vi "Test Customer Pick Up Order Broadcasts Status Update.vi"(8 "error in (no error)":errorcluster, 11 "Customer Test in":refnum<class "Customer Test.lvclass">) -> (0 "error out":errorcluster, 3 "Customer Test out":refnum<class "Customer Test.lvclass">)   [LabVIEW 2020, in "Customer Test.lvclass"]
uses:
  Customer Test.lvclass
  C:/Program Files (x86)/National Instruments/LabVIEW 2020/vi.lib/Asteme/LUnit/Test Case.lvclass
  Processes/People/Customers/Customer/Customer.lvclass
  C:/Program Files (x86)/National Instruments/LabVIEW 2020/vi.lib/Asteme/Triarc Framework/Process/Process.lvclass
  Support/Beverages/Beverage/Beverage.lvclass
  <vilib>/Asteme/LUnit/Test Case.lvclass/Test Case.ctl
  <vilib>/Asteme/LUnit/LUnit Assertion Result.lvclass/LUnit Assertion Result.ctl
  <vilib>/Asteme/Triarc Framework/Process/Process.lvclass/Process.ctl
  <vilib>/Asteme/Triarc Framework/Broadcast Event Helpers/Execution timer.vi
  <vilib>/Asteme/LUnit/Palette/Pass If.vi
  <vilib>/Asteme/LUnit/Set Assertion Type.vi
  <vilib>/Asteme/Triarc Framework/Process/Private/SubVIs/Wait for finish.vi
  <vilib>/Asteme/Triarc Framework/Process/Protected/Messaging/Enqueue Message.vi
  <vilib>/Asteme/Triarc Framework/Process/Private/SubVIs/Set Lifecycle State.vi
  <vilib>/Asteme/Triarc Framework/Process/Public/Lifecycle/Get Lifecycle State.vi
  <vilib>/Asteme/LUnit/Palette/Fail.vi
  <vilib>/Asteme/LUnit/Palette/Pass.vi
  <vilib>/Asteme/LUnit/LUnit Write Assertion Type.vi
  <vilib>/Asteme/LUnit/Add test result.vi
  <vilib>/Asteme/LUnit/LUnit Write Passed.vi
  <vilib>/Asteme/LUnit/LUnit Get Test Case.vi
  <vilib>/Asteme/LUnit/Assertion Result/LUnit Get Test Name.vi
  <vilib>/Asteme/LUnit/LUnit Write Message.vi
  <vilib>/Asteme/LUnit/LUnit Write Description.vi
  <vilib>/Asteme/LUnit/Read Test Case Name.vi
  <vilib>/Asteme/Triarc Framework/Broadcast Event Helpers/Dequeue Broadcast Message.vi
  <vilib>/Utility/error.llb/Error Cluster From Error Code.vi
  <vilib>/Asteme/LUnit/LUnit Assertion Result.lvclass
  <vilib>/Asteme/Triarc Framework/Process/Process.lvclass
  <vilib>/Asteme/LUnit/Test Case.lvclass
  <vilib>/Asteme/Triarc Framework/Broadcast Event Helpers/Broadcast Event Helpers.lvlib
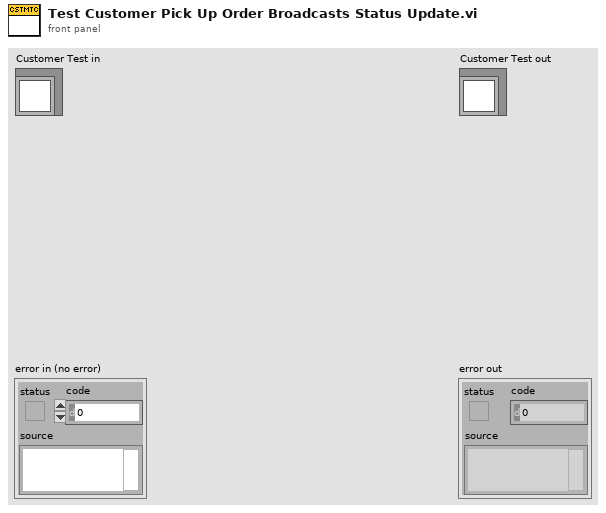
[diagram p1: front panel]
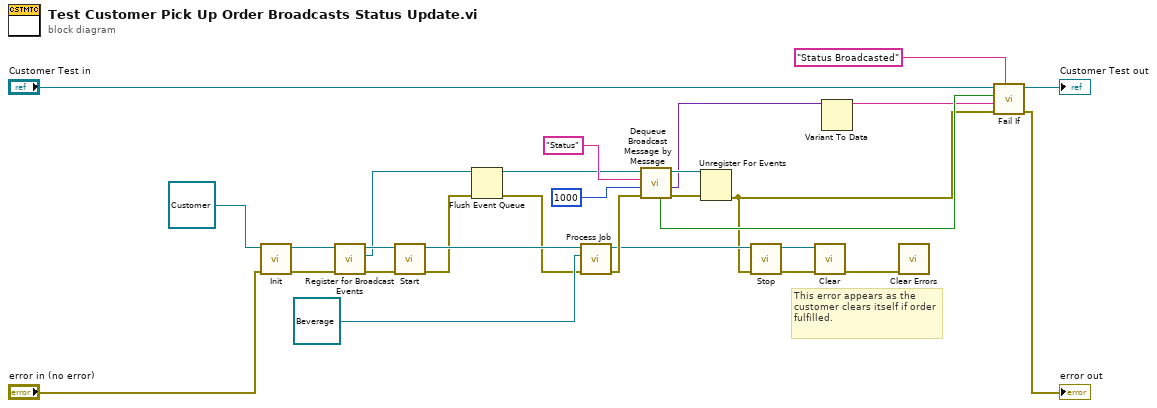
[diagram p0: block diagram]
diagram:
  # "This error appears as the customer clears itself if order fulfilled."
  n1 = call-dynamic "Init.vi"("error in (no error)"="error in (no error)", "View In"=refnum<class "Customer.lvclass"> refnum ("Customer.lvclass")) -> ("error out"=w26:errorcluster, "View Out"=w4:refnum<class "Customer.lvclass">)  [unwired: 8 in]
  n2 = call <vilib>:"Register for Broadcast Events.vi"("error in (no error)"=w26, "Process In"=w4) -> ("error out"=w28:errorcluster, "Event Registration Refnum Out"=w9:refnum<event-registration>, "Process Out"=w27:refnum<class "Customer.lvclass">)  [unwired: 7 in]
  n3 = call <vilib>:"Start.vi"("error in (no error)"=w28, "Process In"=w27) -> ("error out"=w22:errorcluster, "Process Out"=w23:refnum<class "Customer.lvclass">)  [unwired: 8 in]
  n4 = Flush Event Queue(0:w9, 3:w22) -> (8:w8:refnum<event-registration>, 11:w10:errorcluster)  [unwired: 4 in, 1 out]
  n5 = call-dynamic "Process Job.vi"("error in (no error)"=w10, "Job"=refnum<class "Beverage.lvclass"> refnum ("Beverage.lvclass"), "Process Job In"=w23) -> ("error out"=w21:errorcluster, "Process Job Out"=w2:refnum<class "Customer.lvclass">)  [unwired: 7 in]
  n6 = call <vilib>:"Dequeue Broadcast Message by Message.vi"("error in (no error)"=w21, "Timeout (-1)"=1000, "Message"="Status", "Event Registration Refnum"=w8) -> ("error out"=w20:errorcluster, "Message Data"=w6:variant, "Event Registration Refnum Out"=w14:refnum<event-registration>, "Timed Out?"=w7:bool)  [unwired: 3 in, 1 out]
  n7 = Unregister For Events(event registration refnum=w14, error in=w20) -> (error out=w1:errorcluster)
  n8 = call <vilib>:"Stop.vi"("error in (no error)"=w1, "Process In"=w2) -> ("error out"=w25:errorcluster, "Process Out"=w3:refnum<class "Customer.lvclass">)  [unwired: 7 in, 1 out]
  n9 = call-dynamic "Clear.vi"("error in (no error)"=w25, "View In"=w3) -> ("error out"=w17:errorcluster)  [unwired: 9 in]
  n10 = Variant To Data(Variant=w6) -> (data=w5:string)  [unwired: 2 in, 1 out]
  n11 = call <vilib>:"Clear Errors.vi"("error in (no error)"=w17) -> ()  [unwired: 5 in, 2 out]
  n12 = call <vilib>:"Fail If.vi"("Description"="Status Broadcasted", "error in (no error)"=w1, "Message"=w5, "Fail?"=w7, "Test Case In"="Customer Test in") -> ("error out"=→"error out":errorcluster, "Test Case Out"=→"Customer Test out":refnum<class "Customer Test.lvclass">)  [unwired: 5 in]
